vi "get dependency list.vi"(8 "error in":errorcluster, 11 "Shared Library Module editor node in":refnum<class "Shared Library Module editor node.lvclass">) -> (0 "error out":errorcluster, 2 "files":T1[](array[typedef]), 3 "Shared Library Module editor node out":refnum<class "Shared Library Module editor node.lvclass">)   [LabVIEW 2013, in "Shared Library Module editor node.lvclass"]
uses:
  Shared Library Module editor node.lvclass
  <vilib>/NI/Tag Bus Data Framework/Configuration Editor/Classes/TBM Configuration Node/deployment configuration.ctl
  <vilib>/NI/Tag Bus Data Framework/Configuration Editor/Classes/Module editor node/module editor node.lvclass
  Shared Library Module editor node.lvclass/Shared Library Module editor node.ctl
  <vilib>/NI/TBM Modules/CLFN/configuration/Shared Library Module configuration.lvclass/Shared Library Module configuration.ctl
  <vilib>/NI/TBM Modules/CLFN/configuration/Shared Library Module configuration.lvclass
  <vilib>/NI/Tag Bus Data Framework/Configuration Editor/Classes/TBM Configuration Node/TBM Configuration Node.lvclass
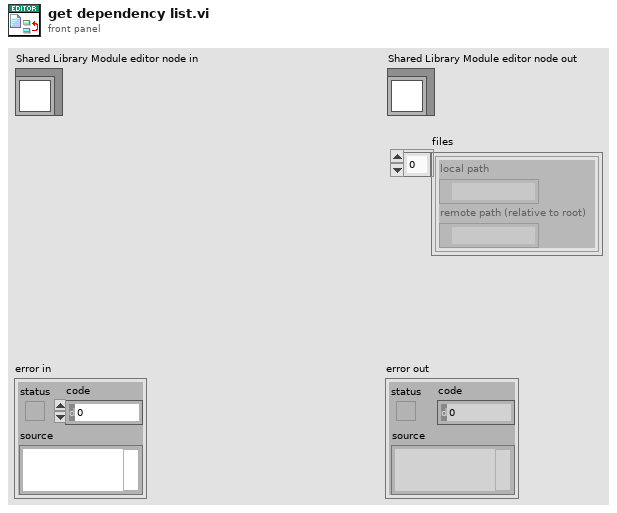
[diagram p1: front panel]
types:
  T1 = typedef "PL Framework Configuration Tool.lvlib/TBM Configuration Node.lvclass/deployment configuration.ctl" = cluster{"local path":path, "remote path (relative to root)":path}
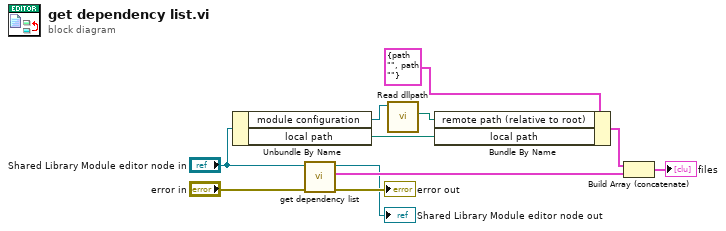
[diagram p0: block diagram]
diagram:
  n1 = Unbundle By Name("Shared Library Module editor node in") -> ("module configuration"=w6:refnum<class "Shared Library Module configuration.lvclass">, "local path"=w2:path)
  n2 = call-parent "get dependency list.vi"("error in"="error in", "TBM Configuration Node in"="Shared Library Module editor node in") -> ("error out"=→"error out":errorcluster, "files"=w10:T1[], "TBM Configuration Node out"=→"Shared Library Module editor node out":refnum<class "Shared Library Module editor node.lvclass">)  [unwired: 7 in]
  n3 = call <vilib>:"Read dllpath.vi"("Shared Library Module configuration in"=w6) -> ("dllpath"=w3:path)  [unwired: 8 in, 2 out]
  n4 = Bundle By Name(cluster=T1 {"local path"=path "", "remote path (relative to root)"=path ""} ("deployment configuration"), "remote path (relative to root)"=w3, "local path"=w2) -> (w1:T1)
  n5 = Build Array (concatenate)(w1, w10) -> (→"files":T1[])
